vi "4p1_HW_Task2B_Doanbs.vi"() -> ()   [LabVIEW 2016]
uses:
  <vilib>/express/express arith-compare/Formula/XNode/ExpressFormulaBlockNode.xnode
panel:
  out "Maximum Range, x":dbl
  out "Maximum Height, y":dbl
  out "Impact Time, t":dbl
  in  "Launch Angle, Theta":dbl
  in  "Launch Velocity, V":dbl
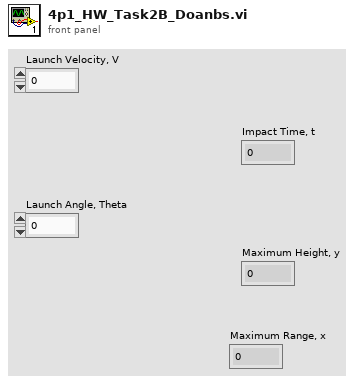
[diagram p1: front panel]
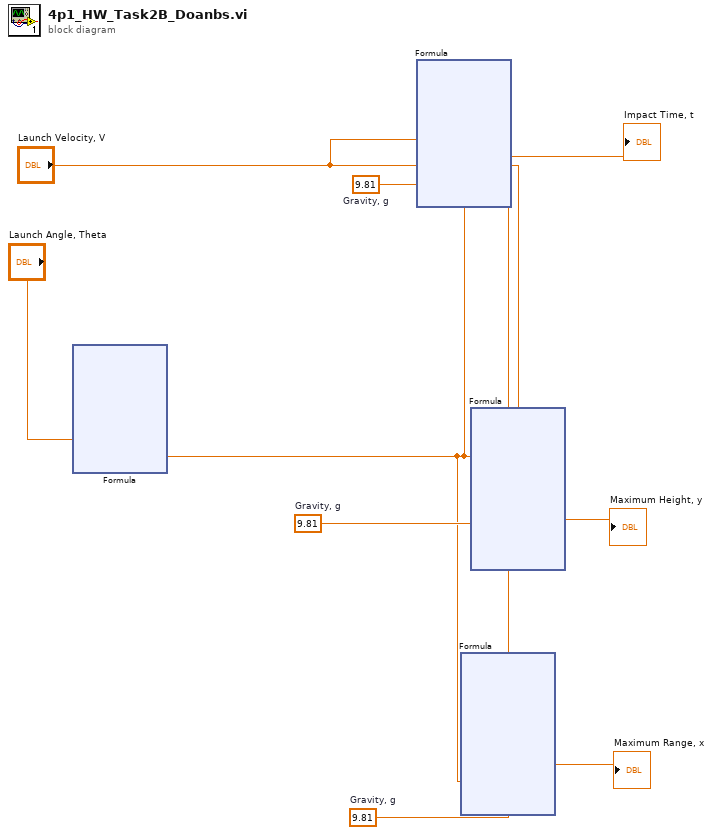
[diagram p0: block diagram]
diagram:
  w4 = 9.81  # Gravity, g
  w7 = 9.81  # Gravity, g
  w8 = 9.81  # Gravity, g
  n1 = xnode "Formula"("Theta"="Launch Angle, Theta") -> ("Result"=w1:dbl)  [unwired: 1 in, 1 out]
  n2 = xnode "Formula"("V"="Launch Velocity, V", "Theta"=w1, "g"=w8) -> ("Result"=→"Impact Time, t":dbl)  [unwired: 1 in, 1 out]
  n3 = xnode "Formula"("V"="Launch Velocity, V", "Theta"=w1, "g"=w4) -> ("Result"=→"Maximum Range, x":dbl)  [unwired: 1 in, 1 out]
  n4 = xnode "Formula"("V"="Launch Velocity, V", "Theta"=w1, "g"=w7) -> ("Result"=→"Maximum Height, y":dbl)  [unwired: 1 in, 1 out]
